vi "RosCommunicationManuelMode.vi"() -> ()   [LabVIEW 2016]
uses:
  <userlib>/ROS for LabVIEW Software/ROS/Code/Console/Servers/ServerSubs/TopicDef.ctl
  <userlib>/ROS for LabVIEW Software/ROS/Code/SubVIs/_ROSDirection.ctl
  <userlib>/ROS for LabVIEW Software/ROS/MessageBuilding/std_msgs/subs/stringScalar.vi
panel:
  out "match substring":string
  out "Reply":string
  in  "stop 2":bool
  out "s? t:f 3":string
  in  "stop":bool
  out "output cluster":T1
  in  "Stop Button":bool
  in  "Start Button":bool
  out "XY Graph":cluster{"X":dbl, "Y":dbl}[](graph)
  out "Robot Speed":dbl(knob) scale=0.0..1.57
  out "Stop":bool
  out "En Marche":bool
  in  "?":bool
  in  "?":bool
  in  "?":bool
  in  "?":bool
  in  "?":bool
  # "Manuel"
  # "Automatique"
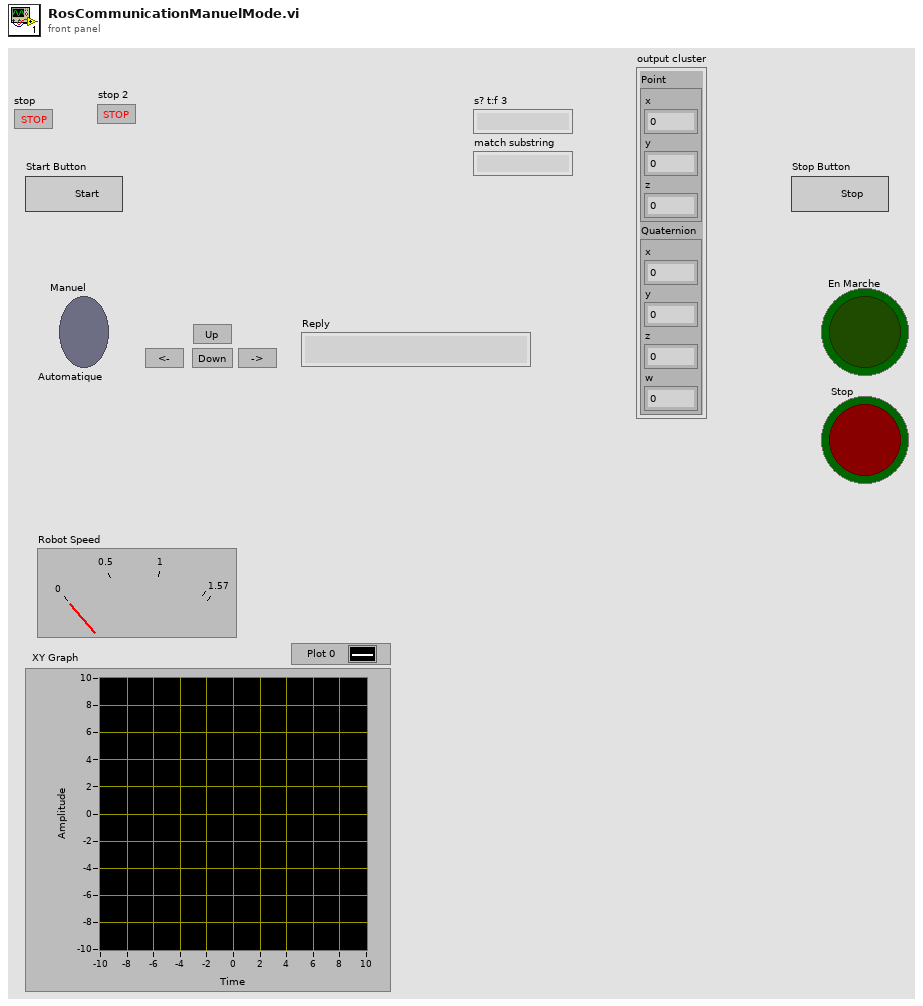
[diagram p1: front panel]
types:
  T1 = cluster{"Point":cluster{"x":dbl, "y":dbl, "z":dbl}, "Quaternion":cluster{"x":dbl, "y":dbl, "z":dbl, "w":dbl}}
  T2 = typedef "TopicDef.ctl" = cluster{"Topic":string, "Type":string, "Action":T3, "Update (ms)":u16, "queue size":u16}
  T3 = typedef "_ROSDirection.ctl" = enum16{"Node", "Publisher", "Subscriber", "ServiceClient", "ServiceProvider"}
  T4 = typedef "_ROSControl.ctl" = cluster{"topic port":u16, "Node":string, "topic":string, "type":string, "node port":u16, "error ":errorcluster, "Direction":T3, "Update (ms)":u16, "FIFO size":u16}
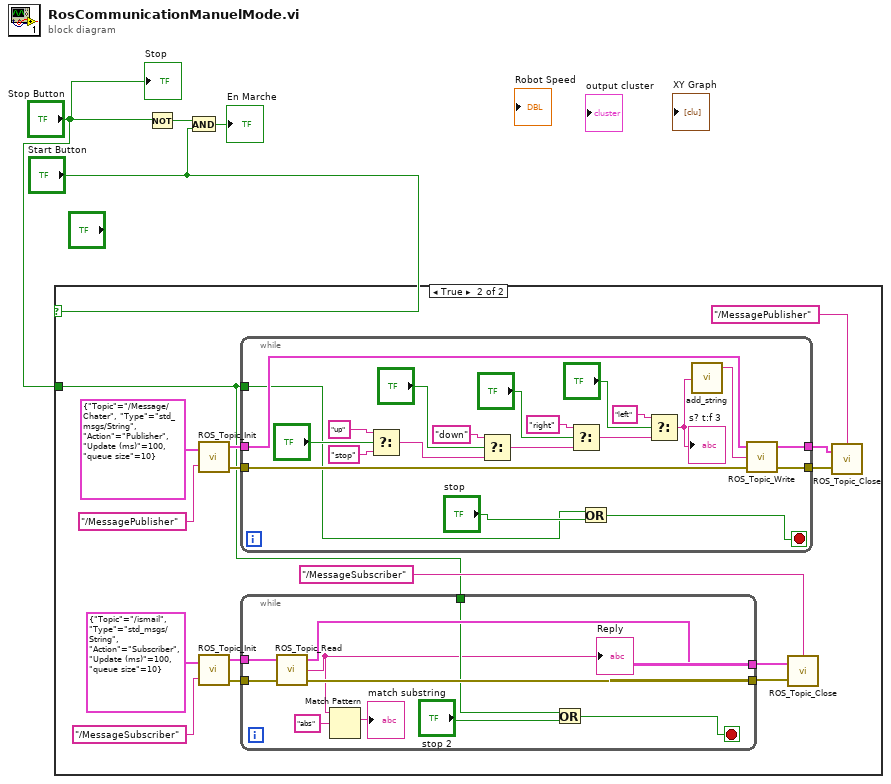
[diagram p0: block diagram]
diagram:
  n1 = case shown="True" "Start Button" {
    tunnel: "Stop Button" -> [_ w5]
    frame False {
    }
    frame True {
      n2 = call <userlib>:"ROS_Topic_Init.vi"("Definitions"=T2 {"Topic"="/Message/Chater", "Type"="std_msgs/String", "Action"=enum."Publisher", "Update (ms)"=100, "queue size"=10}, "node"="/MessagePublisher") -> ("ROS out"=w8:T4, "error out"=w9:errorcluster)  [unwired: 1 in]
      n3 = call <userlib>:"ROS_Topic_Init.vi"("Definitions"=T2 {"Topic"="/ismail", "Type"="std_msgs/String", "Action"=enum."Subscriber", "Update (ms)"=100, "queue size"=10}, "node"="/MessageSubscriber") -> ("ROS out"=w14:T4, "error out"=w13:errorcluster)  [unwired: 1 in]
      n4 = while {
        tunnel: w8 -> [w50]
        tunnel: w9 -> [w49]
        tunnel: [w47] -> w10
        tunnel: [w46] -> w11
        tunnel: w5 -> [w30]
        stop <- w31 stop-if-true
        n5 = Select(t="up", s="?", f="stop") -> (s? t:f=w43:string)
        n6 = Select(t="down", s="?", f=w43) -> (s? t:f=w44:string)
        n7 = Select(t="right", s="?", f=w44) -> (s? t:f=w45:string)
        n8 = Or(x=w30, y="stop") -> (x .or. y?=w31:bool)
        n9 = Select(t="left", s="?", f=w45) -> (s? t:f=w33:string)
        "s? t:f 3" <- w33
        n10 = call-poly <userlib>:"add_string.vi"("String"=w33) -> ("msg out"=w48:string)  [unwired: 4 in]
        n11 = call <userlib>:"ROS_Topic_Write.vi"("error in (no error)"=w49, "Msg in"=w48, "ROS in"=w50) -> ("error out"=w46:errorcluster, "ROS out"=w47:T4)  [unwired: 1 in]
      }
      n12 = while {
        tunnel: w14 -> [w29]
        tunnel: w13 -> [w28]
        tunnel: [w27] -> w18
        tunnel: [w26] -> w19
        tunnel: w5 -> [w23]
        stop <- w25 stop-if-true
        n13 = call <userlib>:"ROS_Topic_Read.vi"("error in (no error)"=w28, "ROS in"=w29) -> ("error out"=w26:errorcluster, "Reply"=w21:string, "ROS out"=w27:T4)  [unwired: 1 in]
        "Reply" <- w21
        n14 = Match Pattern(string=w21, regular expression="abs") -> (match substring=→"match substring":string)  [unwired: 1 in, 3 out]
        n15 = Or(x=w23, y="stop 2") -> (x .or. y?=w25:bool)
      }
      n16 = call <userlib>:"ROS_Topic_Close.vi"("error in"=w19, "ROS in"=w18, "node"="/MessageSubscriber") -> ()  [unwired: 1 in, 1 out]
      n17 = call <userlib>:"ROS_Topic_Close.vi"("error in"=w11, "ROS in"=w10, "node"="/MessagePublisher") -> ()  [unwired: 1 in, 1 out]
    }
  }
  n18 = Not(x="Stop Button") -> (.not. x?=w4:bool)
  n19 = And(x=w4, y="Start Button") -> (x .and. y?=→"En Marche":bool)
  "Stop" <- "Stop Button"
